vi "FRCts20_WebMethods_WrongMethod.vi"(5 "Method Inputs":string[](array[string])) -> (2 "error out":errorcluster)   [LabVIEW 2013, in "FRCts20_WebMethods.lvlib"]
doc: "Checks to see if any of the inputs are blank. If so returns an error."
uses:
  FRCts20_WebMethods.lvlib
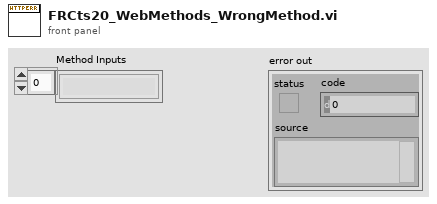
[diagram p1: front panel]
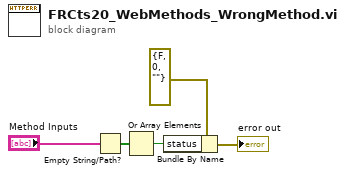
[diagram p0: block diagram]
diagram:
  n1 = Empty String/Path?(string/path="Method Inputs") -> (empty?=w1:bool[])
  n2 = Or Array Elements(Boolean array=w1) -> (logical OR=w4:bool)
  n3 = Bundle By Name(cluster=errorcluster {"status"=FALSE, "code"=0, "source"=""} ("error constant"), "status"=w4) -> (→"error out":errorcluster)
